vi "App Run.vi"(8 "error in (no error)":errorcluster, 10 "Core APIs":T1, 11 "App in":refnum<class "App.lvclass">) -> (0 "error out":errorcluster)   [LabVIEW 2020, in "Volatus.lvlib" / "App.lvclass"]
uses:
  App.lvclass
  Core APIs.ctl
  VolatusAPI/VolatusAPI.lvclass
  App.lvclass/App.ctl
  Volatus.lvlib
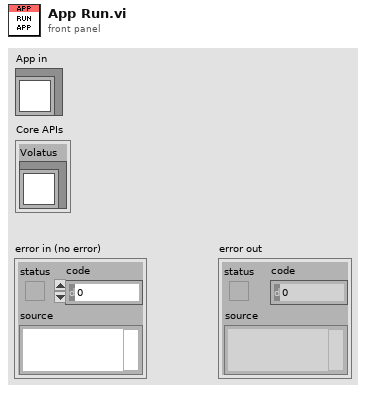
[diagram p1: front panel]
types:
  T1 = typedef "Volatus.lvlib/Core APIs.ctl" = cluster{"Volatus":refnum<class "VolatusAPI.lvclass">}
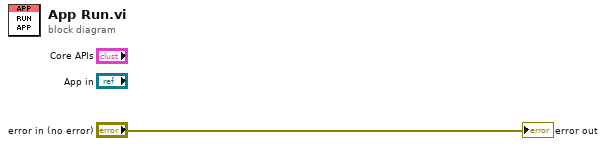
[diagram p0: block diagram]
diagram:
  "error out" <- "error in (no error)"
